vi "Read Standard Event Status.vi"(8 "error in (no error)":errorcluster, 11 "SR3XXX HVPS in":refnum<class "SR3XXX HVPS.lvclass">) -> (0 "error out":errorcluster, 2 "Byte":bool[](array[boolean]), 3 "SR3XXX HVPS out":refnum<class "SR3XXX HVPS.lvclass">)   [LabVIEW 2013, in "SR3XXX HVPS.lvclass"]
doc: "The *ESR common command query reads the value of the standard event status register. If the optional parameter i is present, then only the value of bit i is returned. Reading this register will clear it. Reading bit i will clear bit i only.\n\nBit (Name) Usage\n===========\n0 (OPC) Set by *OPC\n1 unused\n2 (Query Error) Set by an output queue overflow\n3 (Recall Err) Set if a stored setting is corrupt\n4 (Execution Err) Set by an out-of-range parameter or incomplete command.\n5 (Command Err) Set by a command syntax error or an unrecognizable command\n6 (URQ) Set by any key press\n7 (PON) Set by a power-on condition\n\nThis status byte is defined by IEEE488.2 (1987) and is used primarily to report errors in commands received over the communication interface. Once set, the bits in this register stay set, and are cleared when read or when a *CLS command is received. If a bit in the standard status register is set, and the corresponding\nbit in the standard status enable register is set, then the ESB bit in the serial poll register is set."
uses:
  SR3XXX HVPS.lvclass
  Reusable/Session APIs/Serial/Typedefs/Session Handle.ctl
  Reusable/Session APIs/Serial/Serial Session.lvclass
  Base/Session HVPS.lvclass/Session HVPS.ctl
  Base/Read hSession.vi
  Reusable/Session APIs/Serial/Public/Asynchronous Write.vi
  Reusable/Session APIs/Serial/Public/Asynchronous Read.vi
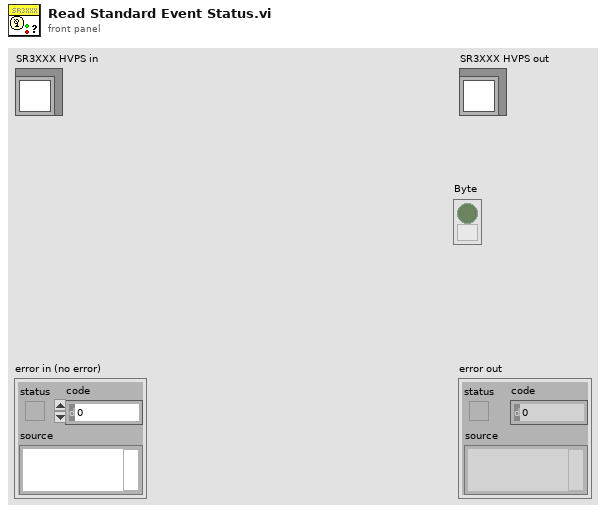
[diagram p1: front panel]
types:
  T1 = typedef "Serial Session.lvclass/Session Handle.ctl" = refnum<data-value>
  T2 = typedef "Session - Root.lvclass/Session Handle.ctl" = refnum<data-value>
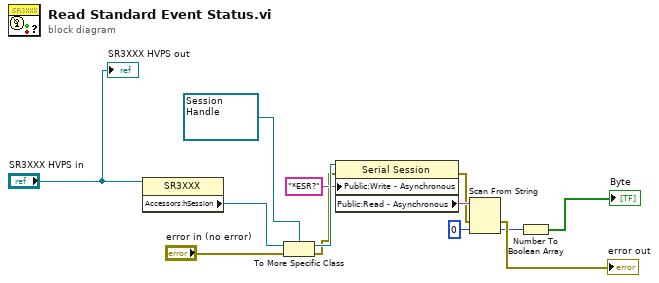
[diagram p0: block diagram]
diagram:
  n1 = property class="SR3XXX"(reference="SR3XXX HVPS in") -> ("Accessors:hSession"=w12:T2)  [unwired: 1 in, 2 out]
  n2 = To More Specific Class(target class=T1 refnum ("Session Handle"), reference=w12, error in="error in (no error)") -> (specific class reference=w10:T1, error out=w6:errorcluster)
  n3 = property class="Serial Session"(reference=w10, error in=w6, "Public:Write - Asynchronous"="*ESR?" ("Cmd")) -> (error out=w5:errorcluster, "Public:Read - Asynchronous"=w8:string)  [unwired: 1 out]
  n4 = Scan From String(input string=w8, error in=w5, default 1=u8 0 ("default value 1")) -> (error out=→"error out":errorcluster, output 1=w2:u8)  [unwired: 2 in, 2 out]
  n5 = Number To Boolean Array(number=w2) -> (Boolean array=→"Byte":bool[])
  "SR3XXX HVPS out" <- "SR3XXX HVPS in"
